vi "Choose heater range.vi"(3 "Heater range mA":string, 8 "error in (no error)":errorcluster, 10 "IP Address in":string="128.174.164.8", 11 "Temp Chan":string="T8") -> (0 "error out":errorcluster, 2 "IP Address out":string)   [LabVIEW 2021]
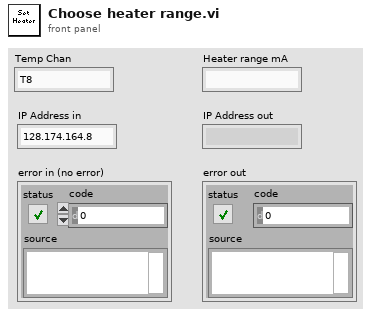
[diagram p1: front panel]
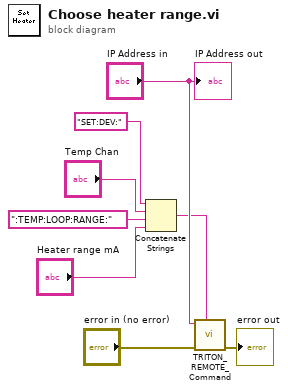
[diagram p0: block diagram]
diagram:
  n1 = Concatenate Strings("SET:DEV:" ("string"), "Temp Chan", ":TEMP:LOOP:RANGE:" ("Command to send"), "Heater range mA") -> (w4:string)
  n2 = call "TRITON_REMOTE_Command.vi"("Command to send"=w4, "error in (no error)"="error in (no error)", "IP Address"="IP Address in") -> ("error out"=→"error out":errorcluster)  [unwired: 6 in, 2 out]
  "IP Address out" <- "IP Address in"
